vi "LoadContainer.vi"(8 "error in (no error)":errorcluster, 11 "Container Path":path) -> (0 "error out":errorcluster)   [LabVIEW 2020, in "VIDiffUtilities.lvlib"]
uses:
  VIDiffUtilities.lvlib
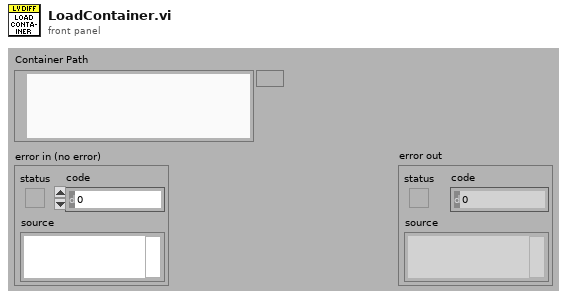
[diagram p1: front panel]
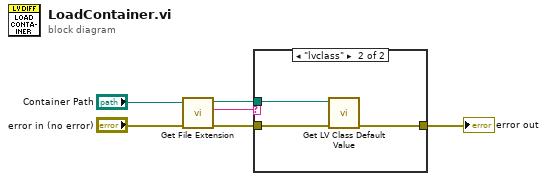
[diagram p0: block diagram]
diagram:
  n1 = call <vilib>:"Get File Extension.vi"("error in (no error)"="error in (no error)", "file"="Container Path") -> ("error out"=w4:errorcluster, "lowercase file extension"=w3:string, "dup file"=w2:path)  [unwired: 5 in, 2 out]
  n2 = case shown="\"lvclass\"" w3 {
    tunnel: w4 -> [w7 w10]
    tunnel: w2 -> [_ w9]
    tunnel: [w7 w8] -> w1
    frame Default {
    }
    frame "lvclass" {
      n3 = call <vilib>:"Get LV Class Default Value.vi"("error in (no error)"=w10, "class path"=w9) -> ("error out"=w8:errorcluster)  [unwired: 8 in, 1 out]
    }
  }
  "error out" <- w1
